vi "Load Controller App.vi"(6 "Open Actor Core front panel? (F)":bool, 8 "Error In":errorcluster, 10 "Mag Lab Measure Controller.lvclass":refnum<class "Mag Lab Measure Controller.lvclass">, 11 "Status Notifier":refnum<notifier>) -> (0 "Error Out":errorcluster)   [LabVIEW 2015, in "Mag Lab Measure Controller.lvclass"]
uses:
  Mag Lab Measure Controller.lvclass
  Mag Lab Measure Controller.lvclass/Mag Lab Measure Controller.ctl
  <vilib>/ActorFramework/Actor/Actor.lvclass
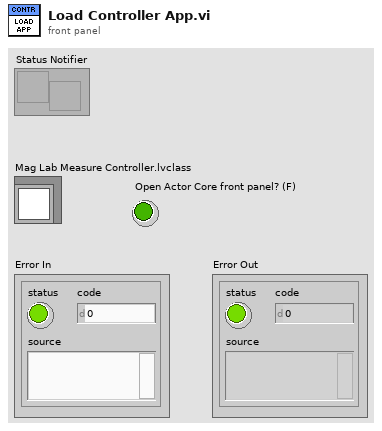
[diagram p1: front panel]
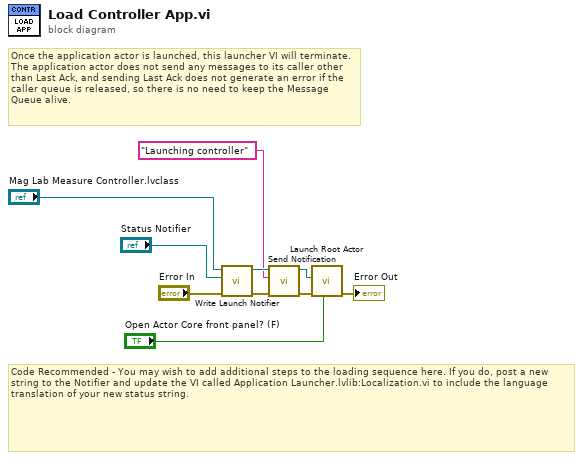
[diagram p0: block diagram]
diagram:
  # "Once the application actor is launched, this launcher VI will terminate. The application actor does not send any messages to its caller other than Last Ack, and sending Last Ack does not generate an error if the caller queue is released, so there is no need to keep the Message Queue alive."
  # "Code Recommended - You may wish to add additional steps to the loading sequence here. If you do, post a new string to the Notifier and update the VI called Application Launcher.lvlib:Localization.vi to include the language translation of your new status string."
  n1 = call "Write Launch Notifier.vi"("error in (no error)"="Error In", "Launch Notifier"="Status Notifier", "Mag Lab Measure Controller in"="Mag Lab Measure Controller.lvclass") -> ("error out"=w3:errorcluster, "Mag Lab Measure Controller out"=w9:refnum<class "Mag Lab Measure Controller.lvclass">)  [unwired: 7 in]
  n2 = call-dynamic "Send Notification.vi"("error in (no error)"=w3, "Notification"="Launching controller" ("notification"), "Mag Lab Measure Controller in"=w9) -> ("error out"=w6:errorcluster, "Mag Lab Measure Controller out"=w4:refnum<class "Mag Lab Measure Controller.lvclass">)  [unwired: 7 in]
  n3 = call <vilib>:"Launch Root Actor.vi"("Open Actor Core front panel? (F)"="Open Actor Core front panel? (F)", "error in (no error)"=w6, "Actor"=w4) -> ("error out"=→"Error Out":errorcluster)  [unwired: 7 in, 1 out]
